vi "TestV5.vi"() -> ()   [LabVIEW 2020]
uses:
  <vilib>/DAQmx/read.llb/DAQmx Read (Analog 2D DBL NChan NSamp).vi
  <vilib>/Analysis/baseanly.llb/Mean (DBL).vi
  <vilib>/DAQmx/miscellaneous.llb/DAQmx Fill In Error Info.vi
  <vilib>/Analysis/NI_AALBase.lvlib
  <resource>/objmgr/daqmx.rc
panel:
  in  "stop":bool
  out "size(s)":i32
  out "Numeric":i32
  out "NumDevices":u32
  out "x/y":dbl
  in  "?":T1(tab)
  in  "Running Module":u8=1 min=1 max=3
  in  "Module 3 Task":refnum<k21>="MyTemperatureTask"
  in  "Sampling Time":u32=5
  in  "Read Time (s)":u32=60
  out "?":dbl[](graph)
  in  "Module 3 File Data Location":path=path "E:/KMUTT/Master Degree/labviewjgsee/log"
  in  "Module 2 File Data Location":path=path "E:/KMUTT/Master Degree/labviewjgsee/log"
  in  "Module 2 Task":refnum<k21>="MyTemperatureTask"
  in  "Module 1 File Data Location":path=path "E:/KMUTT/Master Degree/labviewjgsee/log"
  in  "Module 1 Task":refnum<k21>="MyTemperatureTask"
  in  "DAQmx Device Name":tag
  out "?":string[][](table)
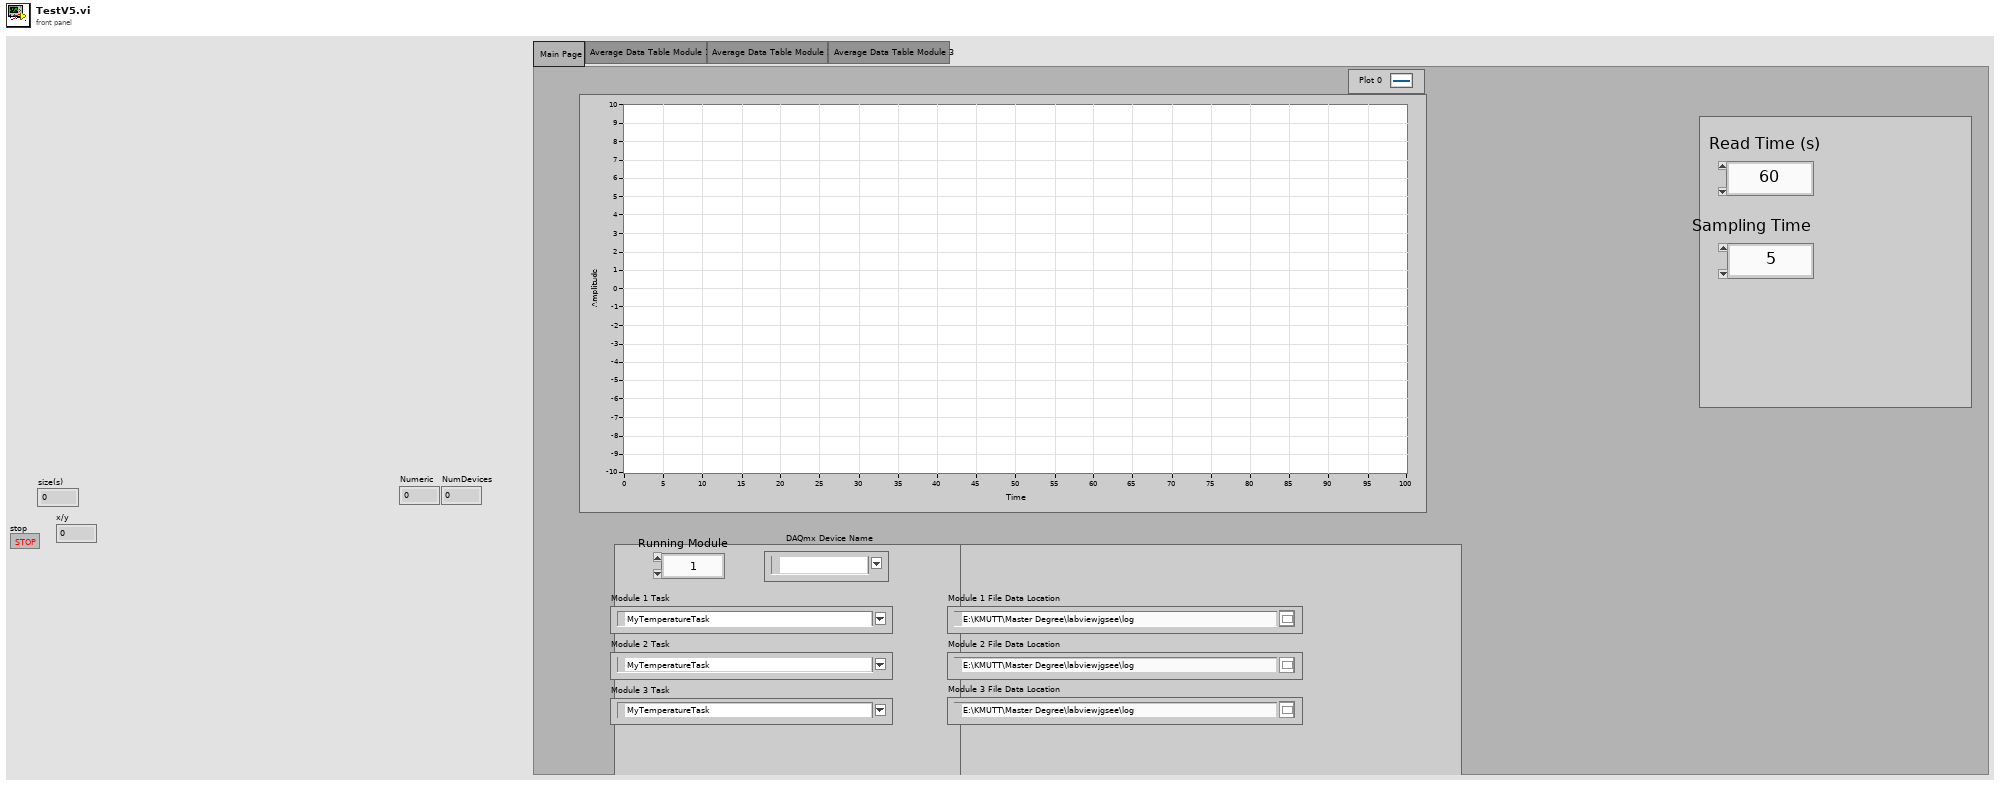
[diagram p1: front panel]
types:
  T1 = enum32{"Main Page ", "Average Data Table Module 1", "Average Data Table Module 2", "Average Data Table Module 3"}
  T2 = enum16{"open", "replace", "create", "open or create", "replace or create", "replace or create with confirmation"}
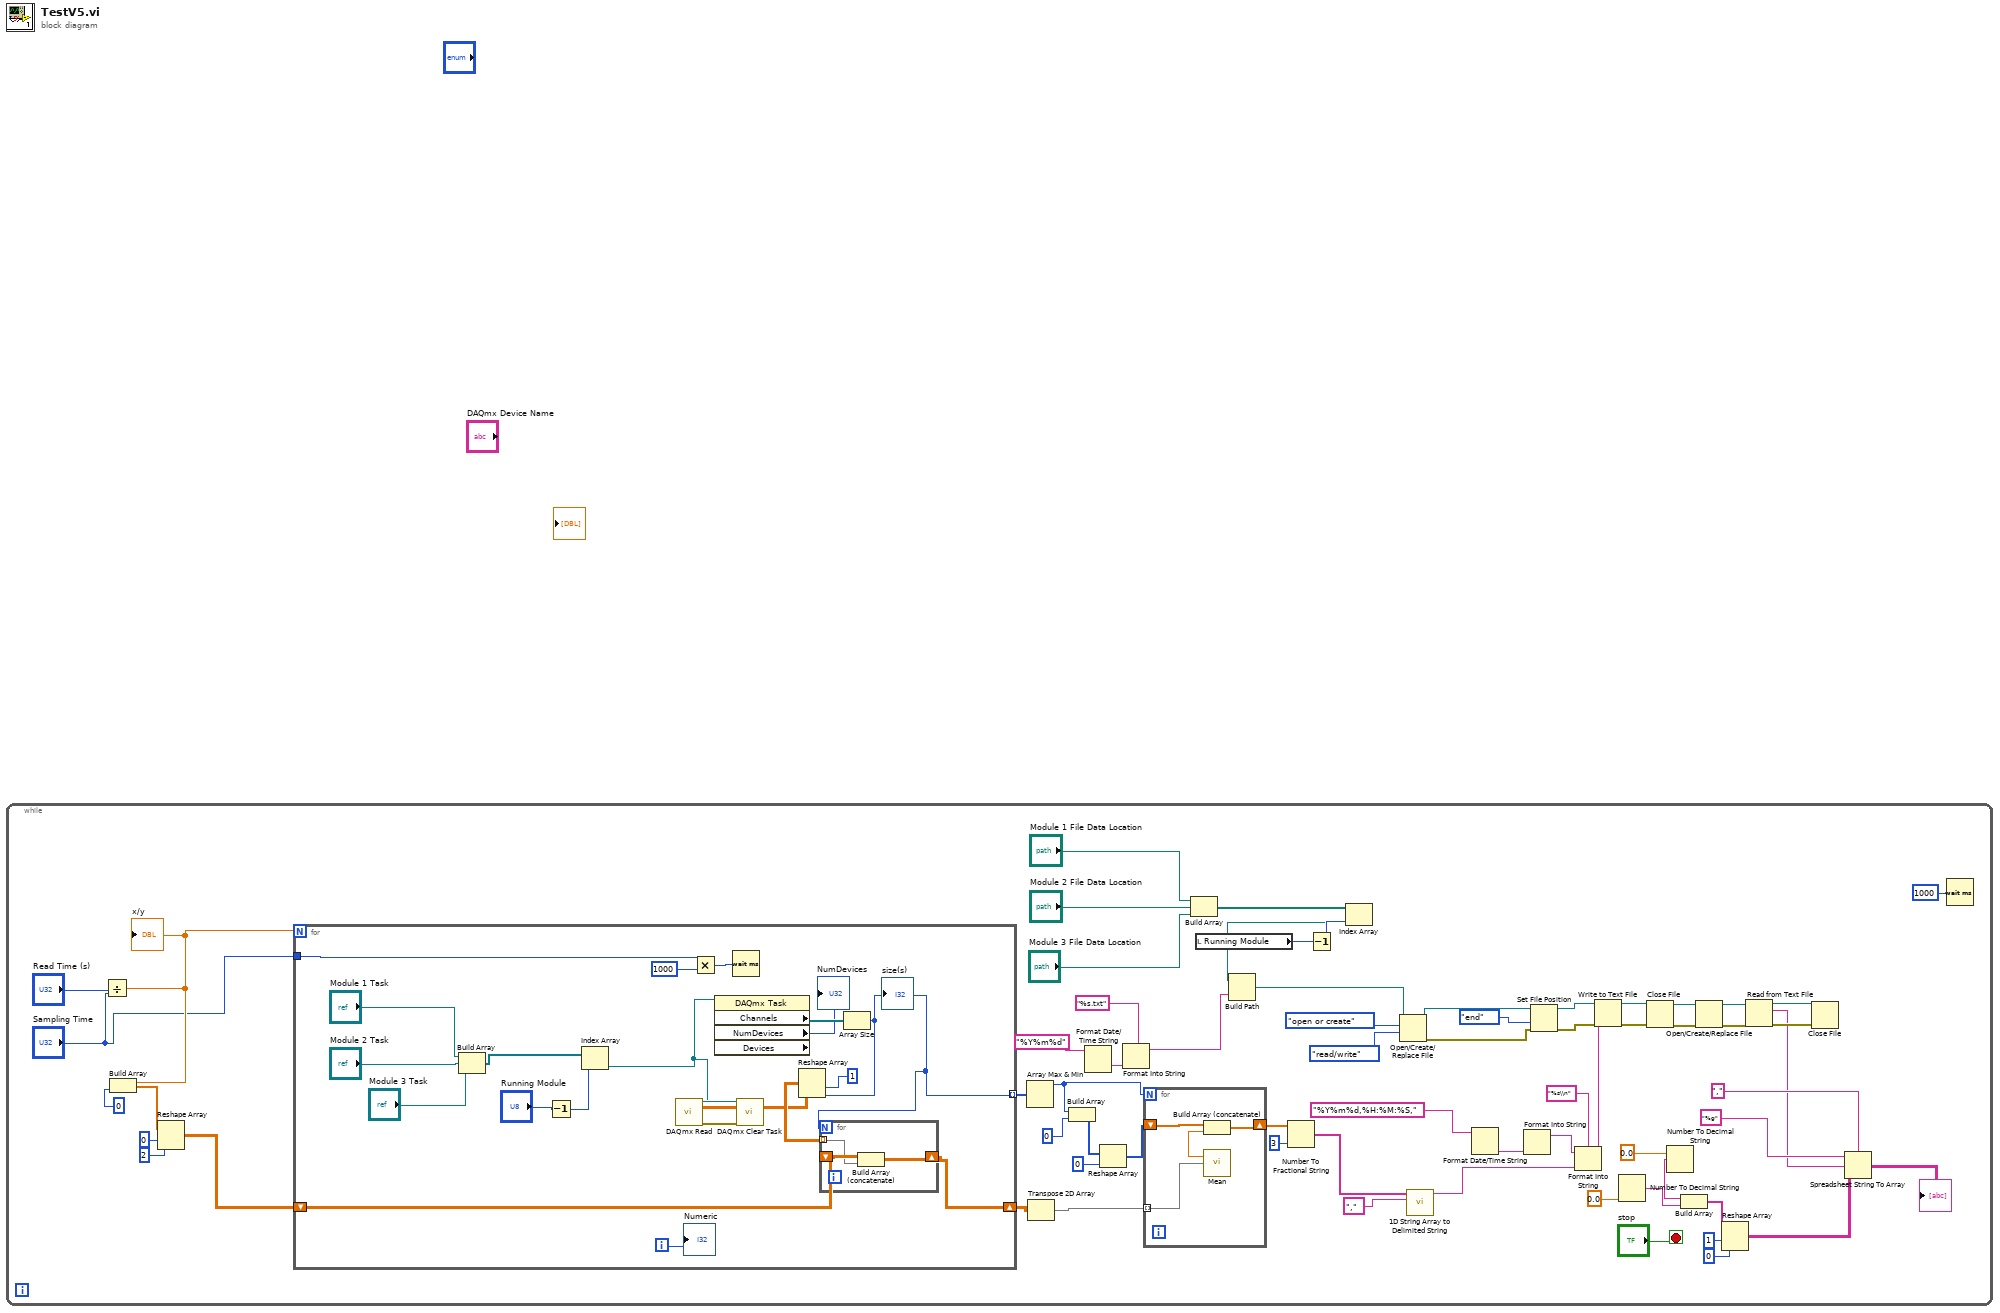
[diagram p0: block diagram]
diagram:
  n1 = while {
    stop <- "stop" stop-if-true
    n2 = Divide(x="Read Time (s)", y="Sampling Time") -> (x/y=w42:dbl)
    "x/y" <- w42
    n3 = Build Array(w42, 0 ("element")) -> (w46:dbl[])
    n4 = Reshape Array(w46, 0 ("dimension size"), 2 ("dimension size")) -> (w43:dbl[][])
    n5 = for {
      N: w42 -> [_]
      shift-right: [w84] -> w11
      shift-left: w43 -> [w83]
      tunnel: "Sampling Time" -> [w82]
      tunnel: [w78] -> w41 mode=indexing
      i -> [w76]
      n6 = Build Array("Module 1 Task", "Module 2 Task", "Module 3 Task") -> (w72:refnum<k21>[])
      n7 = Decrement(x="Running Module") -> (x-1=w68:u8)
      n8 = Index Array(array=w72, index=w68) -> (element=w71:refnum<k21>)
      n9 = call-poly <vilib>:"DAQmx Read.vi"("task/channels in"=w71) -> ("task out"=w87:refnum<k21>, "data"=w77:dbl[][], "error out"=w88:errorcluster)  [unwired: 12 in]
      n10 = Multiply(x=w82, y=u32 1000) -> (x*y=w80:u32)
      n11 = property class="DAQmx Task" props=["Channels", "NumDevices", "Devices"](reference=w71) -> ("Channels"=w79:refnum<k21>[], "NumDevices"=→"NumDevices":u32)  [unwired: 1 in, 3 out]
      n12 = Wait (ms)(milliseconds to wait=w80) -> ()  [unwired: 1 out]
      n13 = call <vilib>:"DAQmx Clear Task.vi"("task in"=w87, "error in"=w88) -> ()  [unwired: 13 in, 1 out]
      n14 = Array Size(array=w79) -> (size(s)=w78:i32)
      "size(s)" <- w78
      n15 = Reshape Array(w77, 1 ("dimension size"), w78) -> (w85:dbl[][])
      n16 = for {
        N: w78 -> [_]
        shift-right: [w90] -> w84
        shift-left: w83 -> [w91]
        tunnel: w85 -> [w89] mode=indexing
        n17 = Build Array (concatenate)(w91, w89) -> (w90:dbl[][])
      }
      "Numeric" <- w76
    }
    n18 = Array Max & Min(array=w41) -> (max value=w38:i32)  [unwired: 3 out]
    n19 = Transpose 2D Array(2D array=w11) -> (transposed array=w40:dbl[][])
    n20 = Build Array(w38, 0 ("element")) -> (w36:i32[])
    n21 = Format Date/Time String(time format string (%c)="%Y%m%d") -> (date/time string=w58:string)  [unwired: 2 in]
    n22 = Reshape Array(w36, 0 ("dimension size")) -> (w35:i32[])
    n23 = Format Into String(format string="%s.txt", w58) -> (resulting string=w56:string)  [unwired: 2 in, 1 out]
    n24 = for {
      N: w38 -> [_]
      tunnel: w40 -> [w95] mode=indexing
      shift-right: [w93] -> w48
      shift-left: w35 -> [w92]
      n25 = call-poly <vilib>:"Mean.vi"("X"=w95) -> ("mean"=w94:dbl)  [unwired: 1 out]
      n26 = Build Array (concatenate)(w92, w94) -> (w93:dbl[])
    }
    n27 = Build Array("Module 1 File Data Location", "Module 2 File Data Location", "Module 3 File Data Location") -> (w3:path[])
    n28 = local read "Running Module"() -> (w4:u8)
    n29 = Number To Fractional String(number=w48, precision (6)=i16 3) -> (F-format string=w49:string[])  [unwired: 2 in]
    n30 = Decrement(x=w4) -> (x-1=w2:u8)
    n31 = Index Array(array=w3, index=w2) -> (element=w1:path)
    n32 = Build Path(base path=w1, name or relative path=w56) -> (appended path=w55:path)
    n33 = Open/Create/Replace File(file path (use dialog)=w55, operation (0:open)=T2."open or create", access (0:read/write)=enum16{"read/write", "read-only", "write-only"}."read/write") -> (refnum out=w33:refnum<file>, error out=w62:errorcluster)  [unwired: 3 in, 1 out]
    n34 = call <vilib>:"1D String Array to Delimited String.vi"("delimiter"="," ("format string"), "string array"=w49) -> ("delimited string"=w54:string)  [unwired: 9 in]
    n35 = Format Date/Time String(time format string (%c)="%Y%m%d,%H:%M:%S,") -> (date/time string=w51:string)  [unwired: 2 in]
    n36 = Format Into String(w51) -> (resulting string=w50:string)  [unwired: 3 in, 1 out]
    n37 = Set File Position(refnum=w33, from (0:start)=enum16{"start", "end", "current"}."end", error in=w62) -> (refnum out=w63:refnum<file>, error out=w61:errorcluster)  [unwired: 1 in]
    n38 = Format Into String(format string="%s\\n", initial string=w50, w54) -> (resulting string=w25:string)  [unwired: 1 in, 1 out]
    n39 = Write to Text File(file (use dialog)=w63, text=w25, error in=w61) -> (refnum out=w32:refnum<file>, error out=w31:errorcluster)  [unwired: 1 in, 1 out]
    n40 = Number To Decimal String(number=0.0 ("element")) -> (decimal integer string=w13:string)  [unwired: 1 in]
    n41 = Close File(refnum=w32, error in=w31) -> (path=w30:path, error out=w29:errorcluster)
    n42 = Number To Decimal String(number=0.0 ("element")) -> (decimal integer string=w15:string)  [unwired: 1 in]
    n43 = Build Array(w15, w13) -> (w17:string[])
    n44 = Open/Create/Replace File(file path (use dialog)=w30, error in=w29) -> (refnum out=w28:refnum<file>, error out=w27:errorcluster)  [unwired: 4 in, 1 out]
    n45 = Reshape Array(w17, 1 ("dimension size"), 0 ("dimension size")) -> (w18:string[][])
    n46 = Read from Text File(file (use dialog)=w28, error in=w27) -> (refnum out=w26:refnum<file>, text=w21:string, error out=w22:errorcluster)  [unwired: 2 in, 1 out]
    n47 = Close File(refnum=w26, error in=w22) -> ()  [unwired: 2 out]
    n48 = Spreadsheet String To Array(delimiter (Tab)=",", format string="%g", spreadsheet string=w21, array type (2D Dbl)=w18) -> (array=→"?":string[][])
    n49 = Wait (ms)(milliseconds to wait=u32 1000) -> ()  [unwired: 1 out]
  }
